vi "BIN_Split_Header_and_content.vi"(8 "error in":errorcluster, 11 "Path in":path) -> (0 "error out":errorcluster, 1 "Content":string, 2 "TAGs":string[](array[string]), 3 "Path out":path, 4 "start of data":i32)   [LabVIEW 2020, in "Sgraph_lib_V1.lvlib" / "DBAL-BIN.lvclass"]
doc: "Read header file portion of Historian Database file"
uses:
  DBAL-BIN.lvclass
  Common/controls/Global-test.vi
  DBAL-BIN.lvclass/DBAL-BIN.ctl
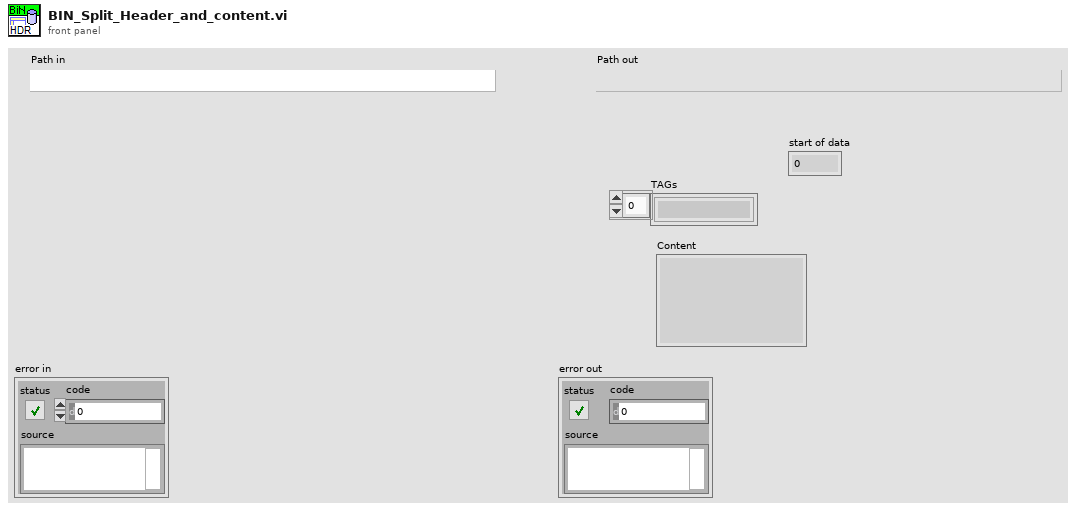
[diagram p1: front panel]
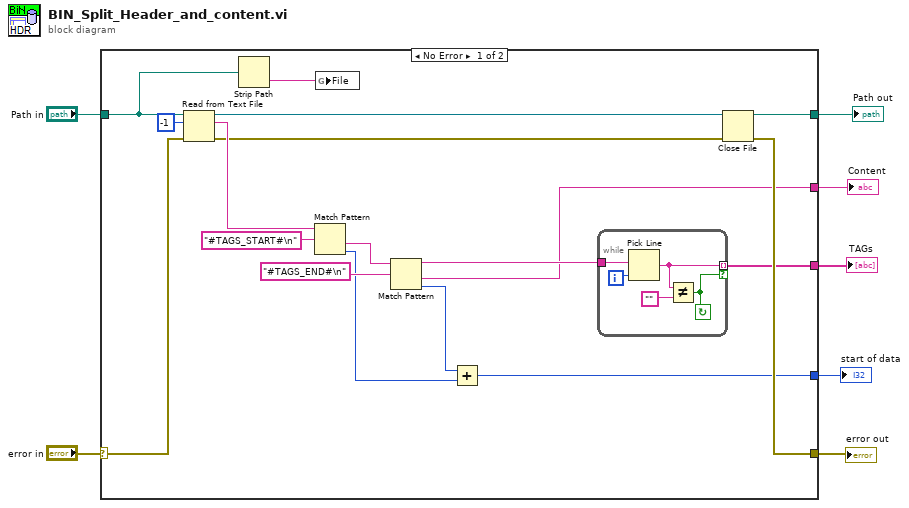
[diagram p0: block diagram]
diagram:
  n1 = case shown="No Error" "error in" {
    selector: "error in" -> [w25 w32]
    tunnel: [w23 w32] -> w6
    tunnel: "Path in" -> [w9 w31]
    tunnel: [w24 w31] -> w4
    tunnel: [w17 _] -> w3
    tunnel: [w14 _] -> w2
    tunnel: [w11 _] -> w1
    frame No Error {
      n2 = Read from Text File(file (use dialog)=w9, count=-1, error in=w25) -> (refnum out=w16:refnum<file>, text=w22:string, error out=w15:errorcluster)  [unwired: 1 in, 1 out]
      n3 = Strip Path(path=w9) -> (name=w8:string)  [unwired: 1 out]
      n4 = Match Pattern(string=w22, regular expression="#TAGS_START#\n") -> (after substring=w20:string, offset past match=w12:i32)  [unwired: 1 in, 2 out]
      n5 = global write "Global-test.vi" "File"(w8) -> ()
      n6 = Match Pattern(string=w20, regular expression="#TAGS_END#\n") -> (before substring=w18:string, after substring=w14:string, offset past match=w13:i32)  [unwired: 1 in, 1 out]
      n7 = Add(x=w13, y=w12) -> (x+y=w11:i32)
      n8 = while {
        tunnel: w18 -> [w26]
        tunnel: [w29] -> w17 mode=indexing if=w27
        i -> [w30]
        stop <- w27 continue-if-true
        n9 = Pick Line(multi-line string=w26, line index=w30) -> (output string=w29:string)  [unwired: 1 in]
        n10 = Not Equal?(x=w29, y="") -> (x != y?=w27:bool)
      }
      n11 = Close File(refnum=w16, error in=w15) -> (path=w24:path, error out=w23:errorcluster)
    }
    frame Error {
    }
  }
  "error out" <- w6
  "Path out" <- w4
  "TAGs" <- w3
  "Content" <- w2
  "start of data" <- w1
